vi "Pre Launch Init.vi"(11 "Main_Control in":refnum<class "Main_Control.lvclass">) -> (0 "error out":errorcluster, 3 "Main_Control out":refnum<class "Main_Control.lvclass">)   [LabVIEW 2021, in "Main_Control.lvlib" / "Main_Control.lvclass"]
doc: "(<B>Filename</B>: Actor Framework.lvlib:Actor.lvclass:Pre Launch Init.vi)\n\nDefines behavior that occurs after the Launch Nested Actor method is invoked but before the actor's Actor Core method begins running.\n\nBy default, this method does nothing. A descendant class may override it to define behavior."
uses:
  Main_Control.lvclass
  Main_Control.lvclass/Main_Control.ctl
  <vilib>/ActorFramework/Actor/Actor.lvclass
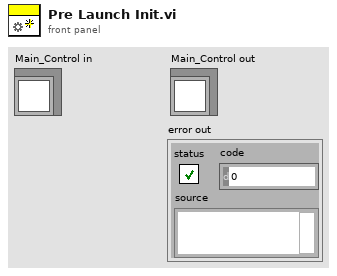
[diagram p1: front panel]
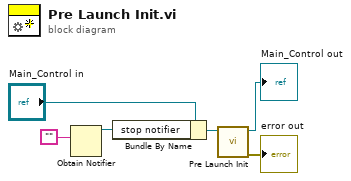
[diagram p0: block diagram]
diagram:
  n1 = Obtain Notifier(notification data type="") -> (notifier out=w3:refnum<notifier>)  [unwired: 3 in, 2 out]
  n2 = Bundle By Name(cluster="Main_Control in", "stop notifier"=w3) -> (w1:refnum<class "Main_Control.lvclass">)
  n3 = call-parent "Pre Launch Init.vi"("Actor in"=w1) -> ("error out"=→"error out":errorcluster, "Actor out"=→"Main_Control out":refnum<class "Main_Control.lvclass">)  [unwired: 9 in]
